vi "create.from_map.vi"(8 "error in":errorcluster, 10 "properties":map{string, string}(c390)) -> (0 "error out":errorcluster, 3 "properties out":refnum<class "properties.lvclass">)   [LabVIEW 2020, in "nominal types.lvlib" / "properties.lvclass"]
uses:
  properties.lvclass
  properties.lvclass/properties.ctl
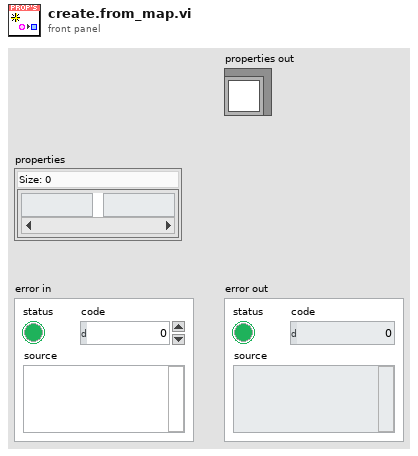
[diagram p1: front panel]
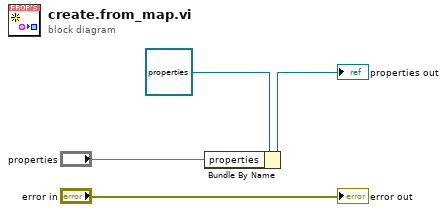
[diagram p0: block diagram]
diagram:
  n1 = Bundle By Name(cluster=refnum<class "properties.lvclass"> refnum ("properties out"), "properties"="properties") -> (→"properties out":refnum<class "properties.lvclass">)
  "error out" <- "error in"
